vi "Read Initialized.vi"(8 "error in (no error)":errorcluster, 11 "device data model in":refnum<class "Device Data Model.lvclass">) -> (0 "error out":errorcluster, 2 "initialized?":bool, 3 "device data model out":refnum<class "Device Data Model.lvclass">)   [LabVIEW 2020, in "SubVIs.lvlib" / "Device Data Model.lvclass"]
uses:
  <vilib>/Modbus/subvis/Data and Functions/Device Data Model/Device Data Model.lvclass
  <vilib>/Modbus/subvis/Data and Functions/Device Data Model/Device Data Model.lvclass/Device Data Model.ctl
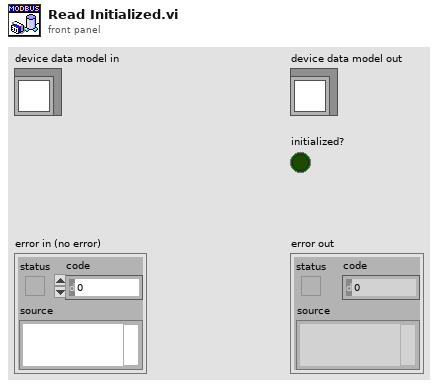
[diagram p1: front panel]
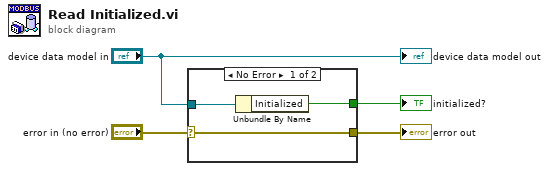
[diagram p0: block diagram]
diagram:
  n1 = case shown="No Error" "error in (no error)" {
    selector: "error in (no error)" -> [w5 w8]
    tunnel: "device data model in" -> [w7 _]
    tunnel: [w6 _] -> w3
    tunnel: [w5 w8] -> w1
    frame No Error {
      n2 = Unbundle By Name(w7) -> ("Initialized"=w6:bool)
    }
    frame Error {
    }
  }
  "error out" <- w1
  "initialized?" <- w3
  "device data model out" <- "device data model in"
